vi "Recursive Remove Contained Empty Folders.vi"(8 "error in (no error)":errorcluster, 11 "Path":path) -> (0 "error out":errorcluster)   [LabVIEW 2017]
uses:
  <userlib>/_OpenG.lib/file/file.llb/Build Path - File Names Array__ogtk.vi
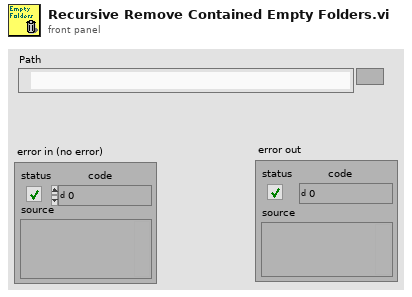
[diagram p1: front panel]
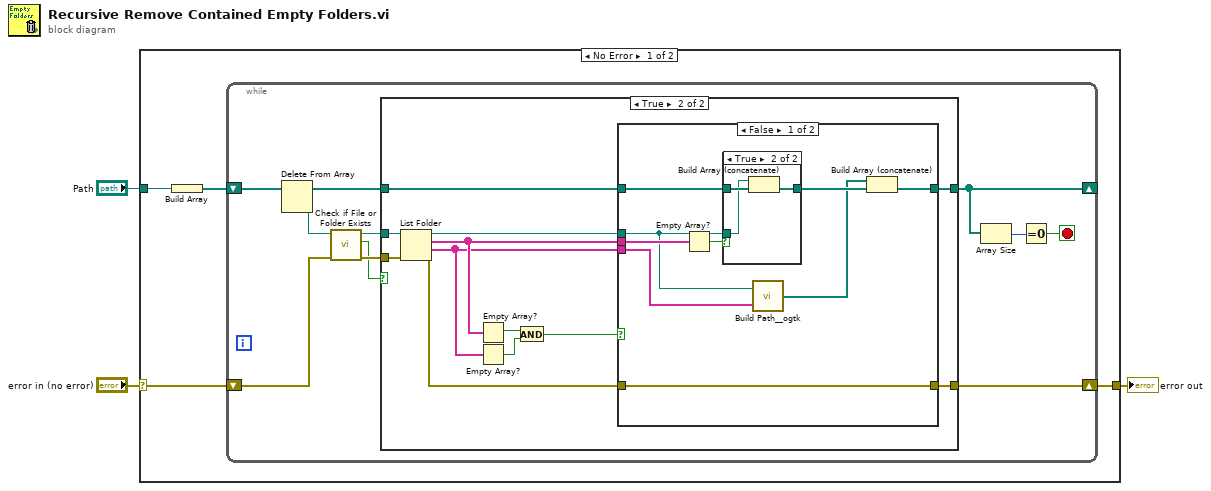
[diagram p0: block diagram]
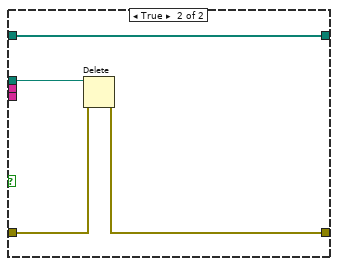
[diagram p4: hidden frame]
diagram:
  n1 = case shown="No Error" "error in (no error)" {
    selector: "error in (no error)" -> [w4 w50]
    tunnel: "Path" -> [w7 _]
    tunnel: [w5 w50] -> w2
    frame No Error {
      n2 = Build Array(w7) -> (w6:path[])
      n3 = while {
        shift-right: [w13] -> _
        shift-left: w6 -> [w18]
        shift-right: [w14] -> w5
        shift-left: w4 -> [w9]
        stop <- w15 stop-if-true
        n4 = Delete From Array(array=w18) -> (deleted portion=w17:path, array with subset deleted=w12:path[])  [unwired: 2 in]
        n5 = call <vilib>:"Check if File or Folder Exists.vi"("error in (no error)"=w9, "path"=w17) -> ("error out"=w10:errorcluster, "file or folder exists?"=w8:bool, "dup path"=w11:path)  [unwired: 7 in]
        n6 = case shown="True" w8 {
          tunnel: [w19 w30] -> w14
          tunnel: [w20 w27] -> w13
          tunnel: w12 -> [w20 w26]
          tunnel: w11 -> [_ w22]
          tunnel: w10 -> [w19 w21]
          frame False {
          }
          frame True {
            n7 = List Folder(path=w22, error in=w21) -> (path out=w31:path, filenames=w25:string[], folder names=w24:string[], error out=w23:errorcluster)  [unwired: 2 in]
            n8 = Empty Array?(array=w25) -> (empty?=w28:bool)
            n9 = Empty Array?(array=w24) -> (empty?=w32:bool)
            n10 = And(x=w28, y=w32) -> (x .and. y?=w29:bool)
            n11 = case shown="False" w29 {
              tunnel: w31 -> [w35 w49]
              tunnel: [w33 w48] -> w30
              tunnel: [w37 w47] -> w27
              tunnel: w26 -> [w40 w47]
              tunnel: w25 -> [w41 _]
              tunnel: w24 -> [w36 _]
              tunnel: w23 -> [w33 w46]
              frame False {
                n12 = Empty Array?(array=w41) -> (empty?=w39:bool)
                n13 = case shown="True" w39 {
                  tunnel: w40 -> [w42 w45]
                  tunnel: [w42 w44] -> w38
                  tunnel: w35 -> [_ w43]
                  frame False {
                  }
                  frame True {
                    n14 = Build Array (concatenate)(w43, w45) -> (w44:path[])
                  }
                }
                n15 = call-poly <userlib>:"Build Path__ogtk.vi"("name or relative path"=w36, "base path"=w35) -> ("appended path"=w34:path[])
                n16 = Build Array (concatenate)(w34, w38) -> (w37:path[])
              }
              frame True {
                n17 = Delete(path (use dialog)=w49, error in=w46) -> (error out=w48:errorcluster)  [unwired: 3 in, 2 out]
              }
            }
          }
        }
        n18 = Array Size(array=w13) -> (size(s)=w16:i32)
        n19 = Equal To 0?(x=w16) -> (x = 0?=w15:bool)
      }
    }
    frame Error {
    }
  }
  "error out" <- w2
